vi "Build Direction Array from Pair.vi"(9 "Pos-Key Map Out":map{T1, string}(c390), 10 "Key-Pos Map Out":map{string, T1}(c390), 11 "output cluster":T2) -> (3 "Direction Array":string[](array[string]))   [LabVIEW 2024]
uses:
  Cluster_Start-End Keys.ctl
  Utility/Universal Utility/TypeDefs_Utility/Cluster_Row-Column.ctl
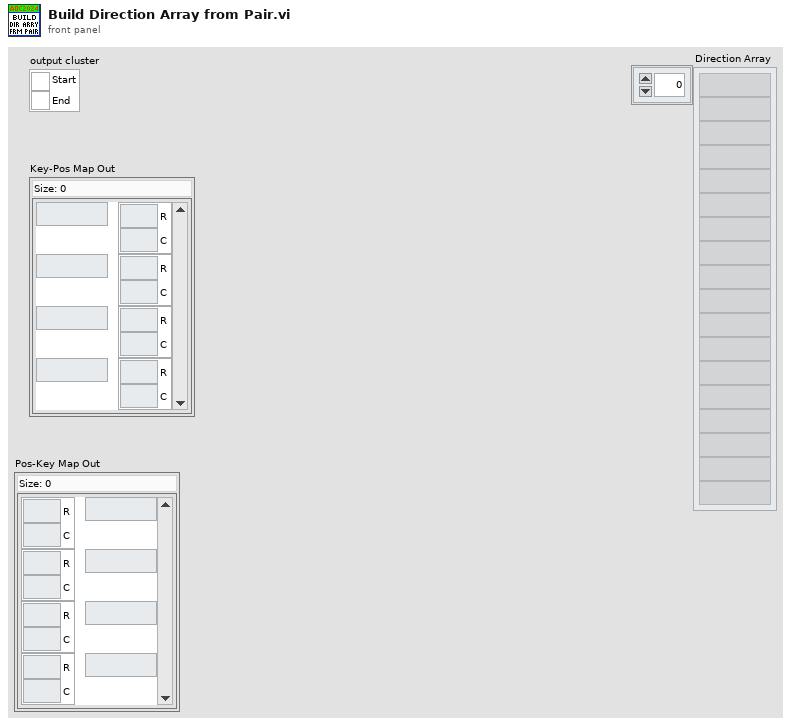
[diagram p1: front panel]
types:
  T1 = typedef "Cluster_Row-Column.ctl" = cluster{"R":i32, "C":i32}
  T2 = typedef "Cluster_Start-End Keys.ctl" = cluster{"Start":string, "End":string}
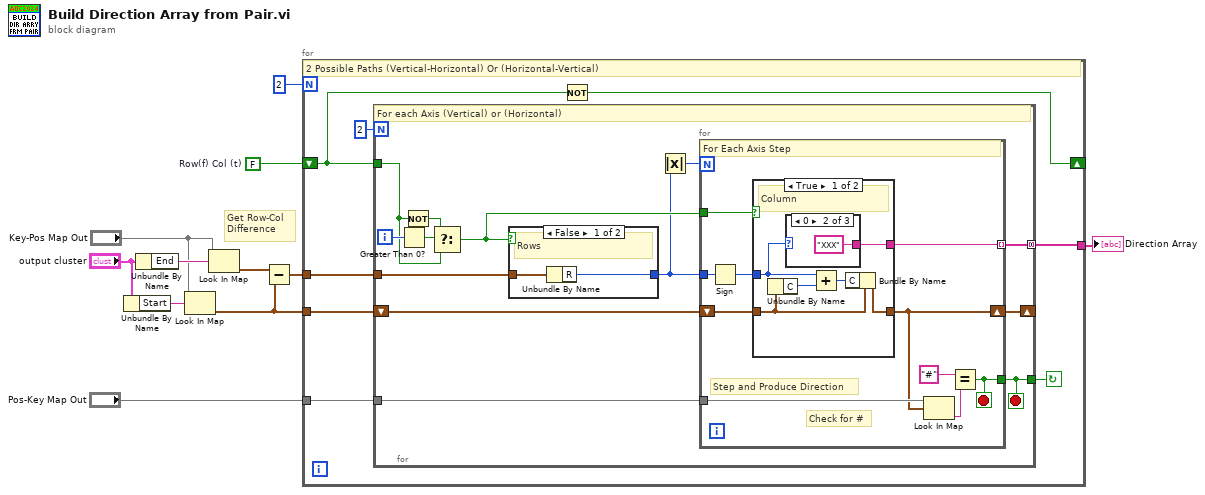
[diagram p0: block diagram]
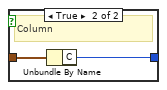
[diagram p2: hidden frame]
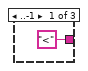
[diagram p3: hidden frame]
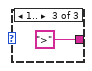
[diagram p4: hidden frame]
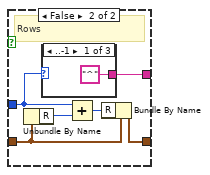
[diagram p5: hidden frame]
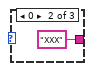
[diagram p6: hidden frame]
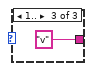
[diagram p7: hidden frame]
diagram:
  w9 = FALSE  # Row(f) Col (t)
  # "Get Row-Col\nDifference"
  n1 = Unbundle By Name("output cluster") -> ("Start"=w2:string)
  n2 = Unbundle By Name("output cluster") -> ("End"=w3:string)
  n3 = Look In Map(map="Key-Pos Map Out", key=w2) -> (value=w6:T1)  [unwired: 1 in, 1 out]
  n4 = Look In Map(map="Key-Pos Map Out", key=w3) -> (value=w4:T1)  [unwired: 1 in, 1 out]
  n5 = Subtract(x=w4, y=w6) -> (x-y=w5:T1)
  n6 = for {
    N: 2 -> [_]
    tunnel: w5 -> [w19]
    tunnel: w6 -> [w17]
    tunnel: "Pos-Key Map Out" -> [w16]
    shift-right: [w14] -> _
    shift-left: w9 -> [w15]
    tunnel: [w12] -> w10
    stop <- w13 continue-if-true
    # "2 Possible Paths (Vertical-Horizontal) Or (Horizontal-Vertical)"
    n7 = for {
      N: 2 -> [_]
      tunnel: w19 -> [w32]
      shift-right: [w22] -> _
      shift-left: w17 -> [w30]
      tunnel: w16 -> [w29]
      tunnel: w15 -> [w25]
      tunnel: [w23] -> w13
      tunnel: [w21] -> w12 mode=concatenating
      i -> [w28]
      stop <- w23 stop-if-true
      # "For each Axis (Vertical) or (Horizontal)"
      n8 = Greater Than 0?(x=w28) -> (x > 0?=w27:bool)
      n9 = Not(x=w25) -> (.not. x?=w26:bool)
      n10 = Select(t=w26, s=w27, f=w25) -> (s? t:f=w24:bool)
      n11 = case shown="False" w24 {
        tunnel: w32 -> [w34 w36]
        tunnel: [w33 w35] -> w20
        frame False {
          # "Rows"
          n12 = Unbundle By Name(w34) -> ("R"=w33:i32)
        }
        frame True {
          # "Column"
          n13 = Unbundle By Name(w36) -> ("C"=w35:i32)
        }
      }
      n14 = Absolute Value(x=w20) -> (abs(x)=w31:i32)
      n15 = for {
        N: w31 -> [_]
        tunnel: w20 -> [w46]
        tunnel: w24 -> [w45]
        tunnel: w29 -> [w41]
        tunnel: [w42] -> w21 mode=indexing
        tunnel: [w37] -> w23
        shift-right: [w39] -> w22
        shift-left: w30 -> [w44]
        stop <- w37 stop-if-true
        # "Check for #"
        # "Step and Produce Direction"
        # "For Each Axis Step"
        n16 = Sign(1:w46) -> (0:w43:i32)
        n17 = case shown="True" w45 {
          tunnel: w44 -> [w52 w61]
          tunnel: w43 -> [w48 w57]
          tunnel: [w49 w58] -> w39
          tunnel: [w47 w56] -> w42
          frame True {
            # "Column"
            n18 = Unbundle By Name(w52) -> ("C"=w51:i32)
            n19 = case shown="0" w48 {
              tunnel: ["<" "XXX" ">"] -> w47
              frame ..-1 {
              }
              frame 0 {
              }
              frame 1.. {
              }
            }
            n20 = Add(x=w48, y=w51) -> (x+y=w50:i32)
            n21 = Bundle By Name(cluster=w52, "C"=w50) -> (w49:T1)
          }
          frame False {
            # "Rows"
            n22 = Unbundle By Name(w61) -> ("R"=w60:i32)
            n23 = case shown="..-1" w57 {
              tunnel: ["^" "XXX" "v"] -> w56
              frame ..-1 {
              }
              frame 0 {
              }
              frame 1.. {
              }
            }
            n24 = Add(x=w57, y=w60) -> (x+y=w59:i32)
            n25 = Bundle By Name(cluster=w61, "R"=w59) -> (w58:T1)
          }
        }
        n26 = Look In Map(map=w41, key=w39) -> (value=w38:string)  [unwired: 1 in, 1 out]
        n27 = Equal?(x="#", y=w38) -> (x = y?=w37:bool)
      }
    }
    n28 = Not(x=w15) -> (.not. x?=w14:bool)
  }
  "Direction Array" <- w10
